vi "Signal Aquisition.vi"() -> (0 "Clap":cluster{"Clap":bool})   [LabVIEW 2015]
uses:
  <vilib>/express/express analysis/Spectral/Block/exnSpectralBlock spectral measurements peak poly.vi
  <vilib>/express/express analysis/Spectral/Block/exnSpectralBlock spectral measurements peak DDT.vi
  <vilib>/imath/engines/lvmath2/RunTimeEngine/Managers/WorkSpace/UID Generator.vi
  <vilib>/imath/engines/lvmath2/RunTimeEngine/RunTimeType/NIMS_RunTimeType_From StrictType (excl LVString).vi
  <instcachedir>/0/NIMS_RunTimeType_From StrictType (excl LVString)_EB1C38A9BC5048DA9ABDA8F781E54D21.lvgen/NIMS_RunTimeType_From StrictType (excl LVString)_EB1C38A9BC5048DA9ABDA8F781E54D21_000.vi
  <vilib>/imath/engines/lvmath2/RunTimeEngine/RunTimeType/NIMS_RunTimeType_Set Source Original Bool.vi
  <vilib>/imath/engines/lvmath2/RunTimeEngine/LocalVariableDefStatement/MC_LocalVariableDefStatement_Display.vi
  <vilib>/imath/engines/lvmath2/RunTimeEngine/Managers/SymbolTable/Clear UID.vi
  <vilib>/imath/engines/lvmath2/RunTimeEngine/NodeEndStatement/NIMS_NodeEndStatement_Output.vi
  <instcachedir>/0/NIMS_NodeEndStatement_Output_53EC0D466D134D7ABD903AC30B43404B.lvgen/NIMS_NodeEndStatement_Output_53EC0D466D134D7ABD903AC30B43404B_012.vi
  <vilib>/imath/engines/lvmath2/RunTimeEngine/ErrorHandling/NIMS_Finalize Error.vi
  <vilib>/express/express analysis/Spectral/XNode/ExpressSpectralMeasurementsBlockNode.xnode
  <vilib>/imath/engines/lvmath2/RunTimeEngine/Managers/SymbolTable/NIMS_WorkSpace.lvlib
panel:
  out "Tone Measurements 2":cluster{"Amplitude":dbl, "Frequency":dbl}={"Amplitude"=0.0007328017088912845, "Frequency"=1500.027668007786}
  out "Aquired Signal 2":dynamicdata(graph)=[{"t0"=timestamp(3532653842.434423 s since 1904-01-01), "dt"=1.9999999999999998e-05, "Y"=array[7680 elements], "attributes"=variant("NI_ChannelName"=variant(string "Voltage"), "NI_UnitDescription"=variant(string "Volts"))}]
  in  "Input Control 2":cluster{"# of samples":i32, "Rate":dbl}={"# of samples"=10000, "Rate"=50000.0}
  out "Spectral Measurements 2":dynamicdata(graph)=[{"t0"=timestamp(0 s since 1904-01-01), "dt"=5.0, "Y"=array[5000 elements], "attributes"=variant("NI_ChannelName"=variant(string "Voltage (FFT - (Peak))"), "NI_OriginalChannelName"=variant(string "Voltage"), "NI_UnitDescription"=variant(string "Volts"))}]
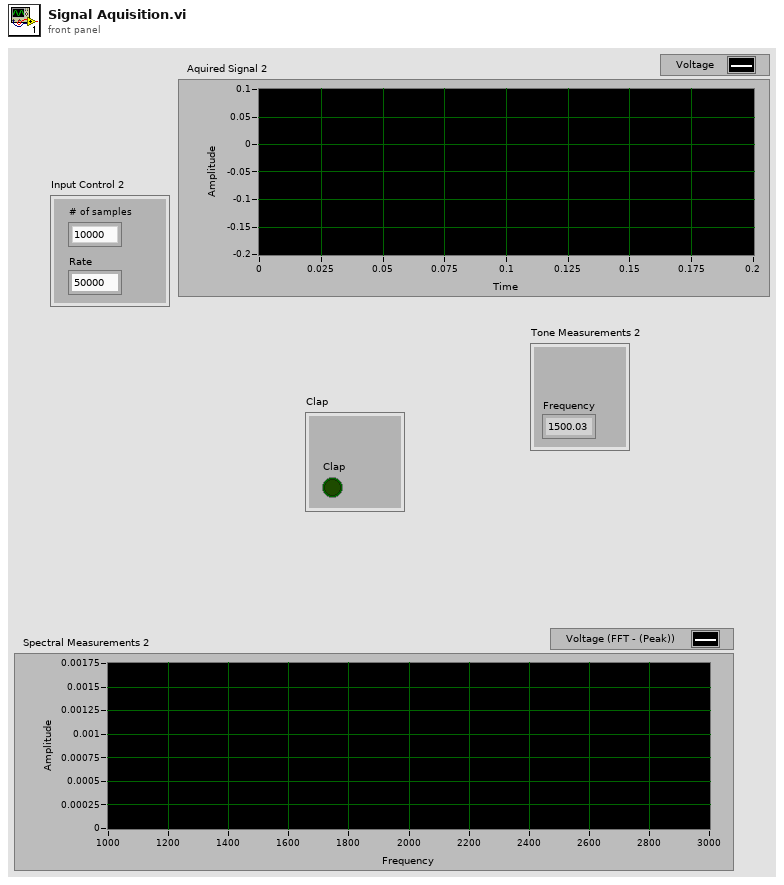
[diagram p1: front panel]
types:
  T1 = cluster{"Amplitude":dynamicdata, "Frequency":dynamicdata}
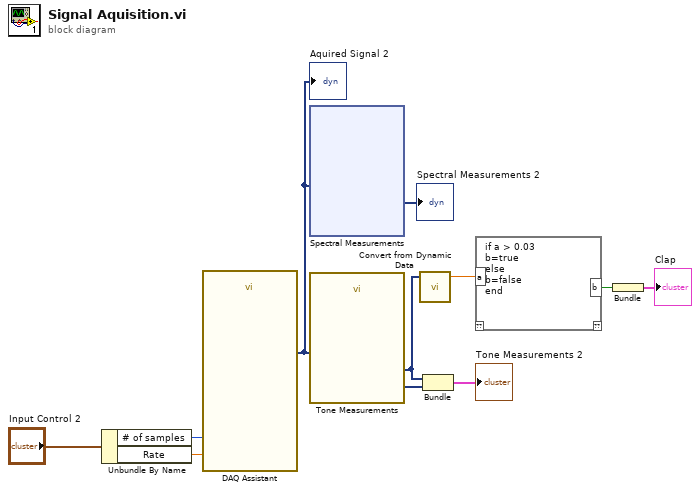
[diagram p0: block diagram]
diagram:
  n1 = Unbundle By Name("Input Control 2") -> ("# of samples"=w2:i32, "Rate"=w1:dbl)
  n2 = call "DAQ Assistant"("rate"=w1, "number of samples"=w2) -> ("data"=w3:dynamicdata)  [unwired: 14 in, 3 out]
  "Aquired Signal 2" <- w3
  n3 = xnode "Spectral Measurements"("Signals"=w3) -> ("FFT - (Peak)"=→"Spectral Measurements 2":dynamicdata)  [unwired: 1 in, 2 out]
  n4 = call "Tone Measurements"("Signals"=w3) -> ("Frequency"=w7:dynamicdata, "Amplitude"=w8:dynamicdata)  [unwired: 8 in, 1 out]
  n5 = call "Convert from Dynamic Data"("Dynamic Data Type"=w8) -> ("Scalar"=w6:dbl)  [unwired: 3 in]
  n6 = Bundle("Amplitude"=w8, "Frequency"=w7) -> (→"Tone Measurements 2":T1)  [unwired: 1 in]
  n7 = mathscript code="if a > 0.03\nb=true\nelse\nb=false\nend"("a"=w6) -> ("b"=w5:bool)  [unwired: 1 in, 1 out]
  n8 = Bundle("b"=w5) -> (→"Clap":cluster{"b":bool})  [unwired: 1 in]
